vi "S_SetProperty.vi"(0 "reference in":refnum<class "SubTemplate_4x4x4.lvclass">, 1 "Property":dbl, 5 "error in (no error)":errorcluster) -> (14 "reference out":refnum<class "SubTemplate_4x4x4.lvclass">, 19 "error out":errorcluster)   [LabVIEW 2020]
uses:
  SubTemplate_4x4x4.lvclass
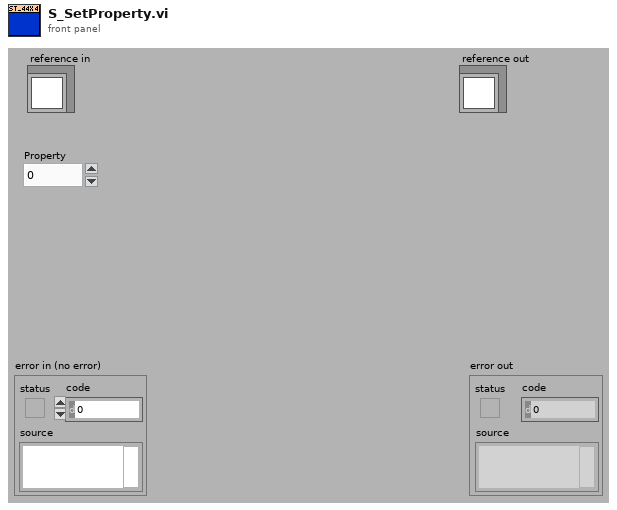
[diagram p1: front panel]
types:
  T1 = typedef "SubTemplate_4x4x4.lvclass/ObjectAttributes.ctl" = cluster{"Base class":T2}
  T2 = typedef "BaseTemplate_4x4x4.lvclass/ObjectAttributes.ctl" = cluster{"Attribute1":dbl}
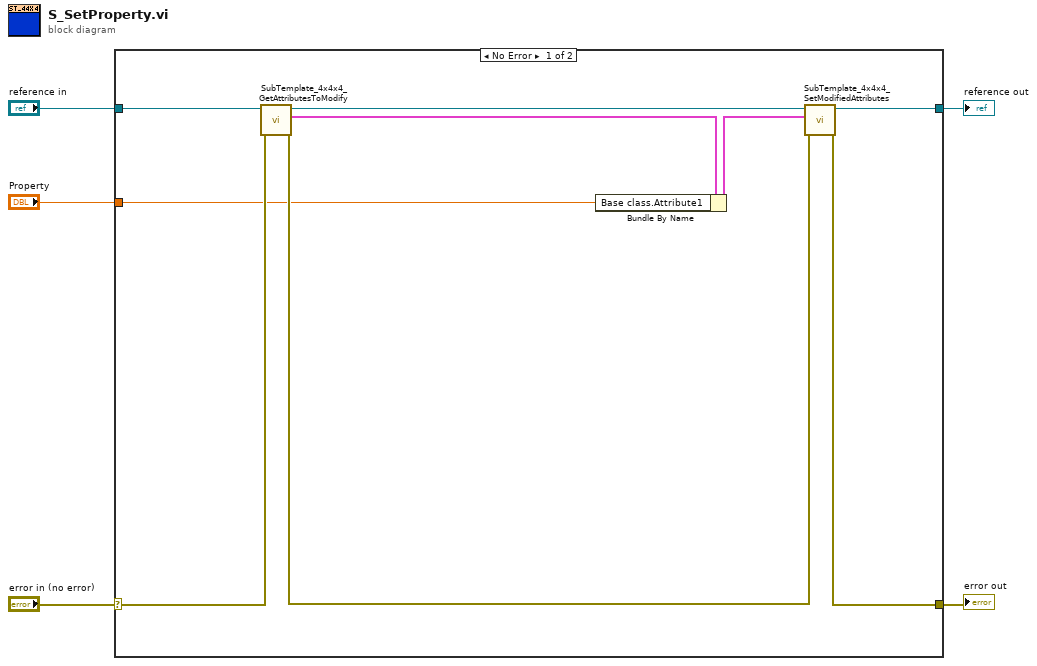
[diagram p0: block diagram]
diagram:
  n1 = case shown="No Error" "error in (no error)" {
    selector: "error in (no error)" -> [w9 w16]
    tunnel: [w11 w16] -> w4
    tunnel: [w8 w15] -> w2
    tunnel: "reference in" -> [w10 w15]
    tunnel: "Property" -> [w6 _]
    frame No Error {
      n2 = call "SubTemplate_4x4x4_GetAttributesToModify.vi"("error in (no error)"=w9, "reference in"=w10) -> ("error out"=w7:errorcluster, "Attributes"=w14:T1, "reference out"=w12:refnum<class "SubTemplate_4x4x4.lvclass">)  [unwired: 6 in, 1 out]
      n3 = Bundle By Name(cluster=w14, "Base class.Attribute1"=w6) -> (w13:T1)
      n4 = call "SubTemplate_4x4x4_SetModifiedAttributes.vi"("error in (no error)"=w7, "Attributes"=w13, "reference in"=w12) -> ("error out"=w11:errorcluster, "reference out"=w8:refnum<class "SubTemplate_4x4x4.lvclass">)  [unwired: 7 in]
    }
    frame Error {
    }
  }
  "error out" <- w4
  "reference out" <- w2
